vi "PSPOP_Show Popup.vi"(6 "Font Size":u32, 7 "Name":string, 8 "error in (no error)":errorcluster, 9 "Call Data (ignore if empty)":variant, 11 "Popup Parameters":T1={"Prop Type"=enum."Unkown", "Initial Value"=variant, "Caption Strings"=[], "Ring Strings"=[], "Cell Rect"={"left"=0, "top"=0, "right"=0, "bottom"=0}, "Mouse Coords"={"x"=0, "y"=0}, "Call Data"=variant, "Ring Values"=[], "Browse Options"={"Prompt"="", "Match Pattern"="", "Mode"=enum."existing file", "Start Path"=path "", "Pattern Label"="", "Button Text"=""}, "Combo Box"={"Allow Undefined Strings"=FALSE}}) -> (0 "error out":errorcluster)   [LabVIEW 2016]
uses:
  Private/Ctrls/POP_Popup Call Parameters.ctl
  Private/Ctrls/POP_Data Type.ctl
  <vilib>/Utility/miscctls.llb/LVBrowseOptionsTypeDef.ctl
  Private/Ctrls/POP_Popup Operation.ctl
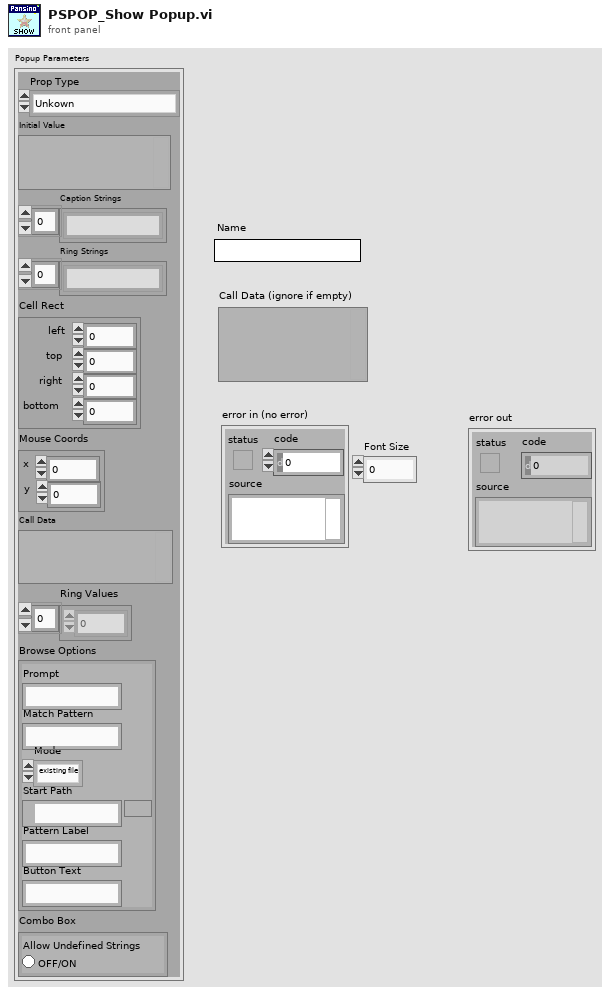
[diagram p1: front panel]
types:
  T1 = typedef "POP_Popup Call Parameters.ctl" = cluster{"Prop Type":T2, "Initial Value":variant, "Caption Strings":string[], "Ring Strings":string[], "Cell Rect":cluster{"left":i16, "top":i16, "right":i16, "bottom":i16}, "Mouse Coords":cluster{"x":i16, "y":i16}, "Call Data":variant, "Ring Values":ext[], "Browse Options":T3, "Combo Box":cluster{"Allow Undefined Strings":bool}}
  T2 = typedef "POP_Data Type.ctl" = enum16{"NO POPUP", "Unkown", "String", "Integer", "Float", "Color", "Boolean", "Ring", "Captioned String", "Captioned Integer", "Button Color", "2 Int Cluster", "4 Int Cluster", "6-Dbl Cluster", "Path", "Combox", "Time", "ShotCut String"}
  T3 = typedef "LVBrowseOptionsTypeDef.ctl" = cluster{"Prompt":string, "Match Pattern":string, "Mode":enum32{"existing file", "new file", "new or existing file", "existing dir", "new dir", "new or existing dir", "existing file (use LLBs)", "new file (use LLBs)", "new or existing file (use LLBs)", "new or existing file or directory (use LLBs)", "existing dir (use LLBs)", "new dir (use LLBs)", "new or existing dir (use LLBs)", "existing file or dir", "new file or dir", "new or existing file or dir", "existing file or dir (use LLBs)", "new file or dir (use LLBs)"}, "Start Path":path, "Pattern Label":string, "Button Text":string}
  T4 = typedef "POP_Popup Operation.ctl" = enum16{"Show", "Initialize", "Close", "Popup Done", "Register a Location's Type", "Retrieve Location's Type"}
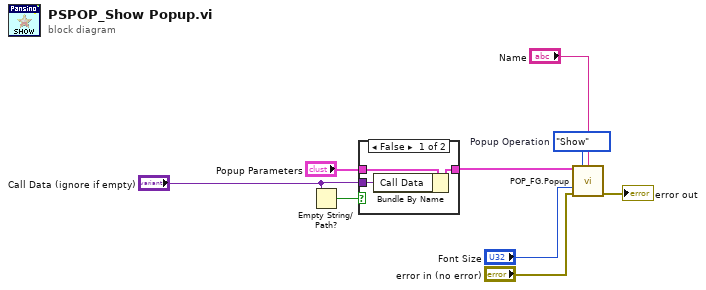
[diagram p0: block diagram]
diagram:
  w9 = POP_Popup_Operation."Show"  # Popup Operation
  n1 = Empty String/Path?(string/path="Call Data (ignore if empty)") -> (empty?=w6:bool)
  n2 = case shown="False" w6 {
    tunnel: "Popup Parameters" -> [w11 w13]
    tunnel: "Call Data (ignore if empty)" -> [w12 _]
    tunnel: [w10 w13] -> w3
    frame False {
      n3 = Bundle By Name(cluster=w11, "Call Data"=w12) -> (w10:T1)
    }
    frame True {
    }
  }
  n4 = call "POP_FG.Popup.vi"("Popup Parameters"=w3, "Popup Operation"=w9, "Name"="Name", "Font Size"="Font Size", "Error In"="error in (no error)") -> ("Error Out"=→"error out":errorcluster)  [unwired: 7 in, 3 out]
